vi "createEventStartupChecks.vi"(8 "error in (no error)":errorcluster, 11 "UserEvents in":refnum<class "UserEvents.lvclass">) -> (0 "error out":errorcluster, 3 "UserEvents out":refnum<class "UserEvents.lvclass">)   [LabVIEW 2016, in "UserEvents.lvclass"]
uses:
  UserEvents.lvclass
  DataTypes/Topics/EventStartupChecks.ctl
  DataTypes/Topics/Parts/Timestamp.ctl
  UserEvents.lvclass/UserEvents.ctl
  DataTypes/Topics/M1M3SupportTopics.lvlib
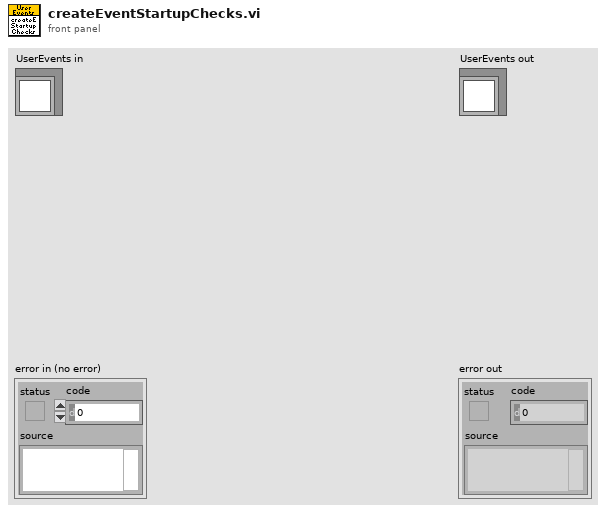
[diagram p1: front panel]
types:
  T1 = typedef "M1M3SupportTopics.lvlib/EventStartupChecks.ctl" = cluster{"Timestamp":T2, "ILCVersionsOk":bool, "DCAVersionsOk":bool, "ILCFirmwareOk":bool, "DCAFirmwareOk":bool, "ILCStatusOk":bool, "DCAStatusOk":bool}
  T2 = typedef "M1M3SupportTopics.lvlib/Timestamp.ctl" = dbl
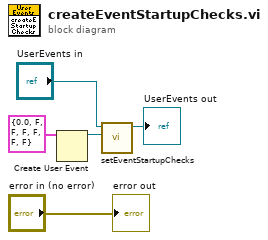
[diagram p0: block diagram]
diagram:
  n1 = Create User Event(user event datatype=T1 {"Timestamp"=0.0, "ILCVersionsOk"=FALSE, "DCAVersionsOk"=FALSE, "ILCFirmwareOk"=FALSE, "DCAFirmwareOk"=FALSE, "ILCStatusOk"=FALSE, "DCAStatusOk"=FALSE} ("EventStartupChecks")) -> (user event=w3:refnum<user-event>)  [unwired: 1 in, 1 out]
  n2 = call "setEventStartupChecks.vi"("EventStartupChecks"=w3, "UserEvents in"="UserEvents in") -> ("UserEvents out"=→"UserEvents out":refnum<class "UserEvents.lvclass">)  [unwired: 9 in]
  "error out" <- "error in (no error)"
